vi "DAQmx Create Channel (AI-Position-EddyCurrentProxProbe).vi"(0 "task in":refnum<k21>, 1 "maximum value":dbl=0.00254 format="%.5f", 2 "minimum value":dbl format="%0.2f", 5 "physical channels":tag, 7 "name to assign":string, 9 "units":i32(ring)=10219 items=["Meters"=10219, "Inches"=10379, "From Custom Scale"=10065], 11 "error in":errorcluster, 12 "custom scale name":tag, 13 "sensitivity":dbl=200.0, 14 "sensitivity units":i32(ring)=14836 items=["mVolts/mil"=14836, "Volts/mil"=14837, "mVolts/mMeter"=14838, "Volts/mMeter"=14839, "mVolts/micron"=14840]) -> (4 "task out":refnum<k21>, 15 "error out":errorcluster)   [LabVIEW 2018]
doc: "Creates channel(s) that use an eddy current proximity probe to measure position."
uses:
  nilvaiu.dll
panel:
  # "input limits"
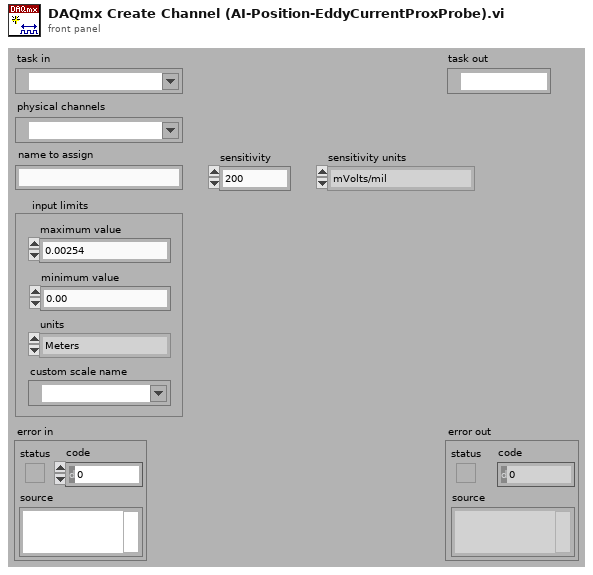
[diagram p1: front panel]
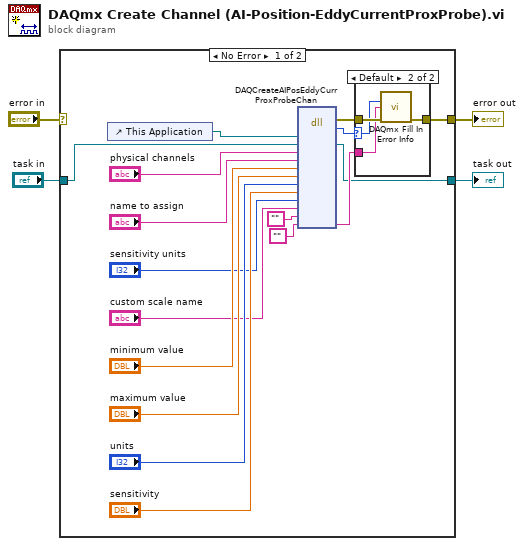
[diagram p0: block diagram]
diagram:
  n1 = case shown="No Error" "error in" {
    selector: "error in" -> [_ w28]
    tunnel: [w16 w28] -> w2
    tunnel: "task in" -> [w14 w27]
    tunnel: [w15 w27] -> w1
    frame No Error {
      n2 = control-ref of="This Application"() -> (w18:refnum<vi>)
      n3 = dll-call lib="nilvaiu.*" fn="DAQCreateAIPosEddyCurrProxProbeChan"("lvAppRef"=w18, "refObjPtr"=w14, "physicalChannelName"="physical channels", "channelNameIn"="name to assign", "minVal"="minimum value", "maxVal"="maximum value", "units"="units", "sensitivity"="sensitivity", "sensitivityUnits"="sensitivity units", "customScaleName"="custom scale name", "channelNamesOut"="", "extendedErrorInfo"="") -> (error out=w21:errorcluster, "return type"=w20:i32, "refObjPtr"=w15:refnum<k21>, "extendedErrorInfo"=w19:string)  [unwired: 13 in, 1 out]
      n4 = case shown="Default" w20 {
        selector: w20 -> [_ w24]
        tunnel: w21 -> [w22 w26]
        tunnel: [w22 w25] -> w16
        tunnel: w19 -> [_ w23]
        frame 0 {
        }
        frame Default {
          n5 = call "DAQmx Fill In Error Info.vi"("status code"=w24, "extended error info"=w23, "error in"=w26) -> ("error out"=w25:errorcluster)  [unwired: 1 in, 11 out]
        }
      }
    }
    frame Error {
    }
  }
  "error out" <- w2
  "task out" <- w1
